vi "Thread.Set Priority.vi"(10 "Priority":i32, 11 "Thread in":refnum<class "Thread.lvclass">) -> (3 "Thread out":refnum<class "Thread.lvclass">)   [LabVIEW 2016, in "Thread.lvclass"]
uses:
  Thread.lvclass
  Thread.lvclass/Thread.ctl
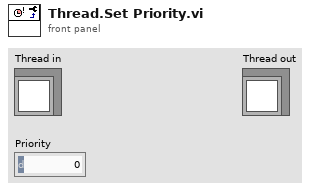
[diagram p1: front panel]
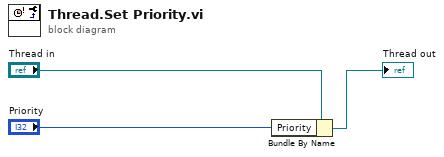
[diagram p0: block diagram]
diagram:
  n1 = Bundle By Name(cluster="Thread in", "Priority"="Priority") -> (→"Thread out":refnum<class "Thread.lvclass">)
